vi "DecodeResponse.vi"(8 "error in (no error)":errorcluster, 11 "data in":string) -> (0 "error out":errorcluster, 3 "RecognitionResponse":T1)   [LabVIEW 2019]
uses:
  RecognitionResponse.ctl
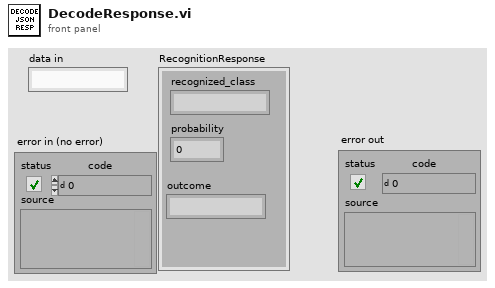
[diagram p1: front panel]
types:
  T1 = typedef "RecognitionResponse.ctl" = cluster{"probability":dbl, "recognized_class":string, "outcome":string}
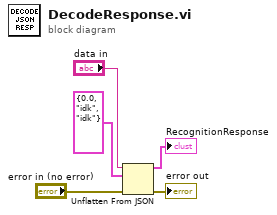
[diagram p0: block diagram]
diagram:
  n1 = Unflatten From JSON(JSON string="data in", type and defaults=T1 {"probability"=0.0, "recognized_class"="idk", "outcome"="idk"} ("RecognitionRequest"), error in (no error)="error in (no error)") -> (value=→"RecognitionResponse":T1, error out=→"error out":errorcluster)  [unwired: 4 in]
